vi "MD5 PaddingU8.vi"(10 "Pre Buffer Size":i64, 11 "Current Buffer":u8[](array[numeric])) -> (3 "MD5 Padded Buffer":u8[](array[numeric]))   [LabVIEW 2009]
doc: "A U8 padding VI for MD5 hash generation"
panel:
  # "[OpenG VI Tags] ***Do Not Remove***"
  # "MD5 Padding.vi\n\nDerived from the RSA Data Security, Inc. MD5 Message-Digest Algorithm\n\nPlease visit http://www.OpenG.org to learn about the\nOpen Source LabVIEW software movement.\n\nNOTICE -- YOU MUST LEAVE THIS NOTICE IN PLACE.  PER THE TERMS OF THE LICENSE BELOW, YOU MAY SUBLICENSE THIS SOFTWARE \nIN ANY WAY THAT DOES NOT CONFLICT WITH THIS LICENSE.\n\n### BSD License (http://www.opensource.org/licenses/bsd-license.php) Begin ###\n \nCopyright (c) 2004, Enrique Vargas <vargas@visecurity.com>\n\nAll rights reserved.\n\nRedistribution and use in source and binary forms, with or without modification, are permitted provided that the following conditions are met:\n\n    * Redistributions of source code must retain the above copyright notice, this list of conditions and the following disclaimer.\n    * Redistributions in binary form must reproduce the above copyright notice, this list of conditions and the following disclaimer in the \n       documentation and/or other materials provided with the distribution.\n    * Neither the name of SciWare, James Kring, Inc., nor the names of its contributors may be used to endorse or promote products derived \n       from this software without specific prior written permission.\n\nTHIS SOFTWARE IS PROVIDED BY THE COPYRIGHT HOLDERS AND CONTRIBUTORS \"AS IS\" AND ANY EXPRESS OR IMPLIED WARRANTIES, \nINCLUDING, BUT NOT LIMITED TO, THE IMPLIED WARRANTIES OF MERCHANTABILITY AND FITNESS FOR A PARTICULAR PURPOSE ARE \nDISCLAIMED. IN NO EVENT SHALL THE COPYRIGHT OWNER OR CONTRIBUTORS BE LIABLE FOR ANY DIRECT, INDIRECT, INCIDENTAL,\n SPECIAL, EXEMPLARY, OR CONSEQUENTIAL DAMAGES (INCLUDING, BUT NOT LIMITED TO, PROCUREMENT OF SUBSTITUTE GOODS OR \nSERVICES; LOSS OF USE, DATA, OR PROFITS; OR BUSINESS INTERRUPTION) HOWEVER CAUSED AND ON ANY THEORY OF LIABILITY, \nWHETHER IN CONTRACT, STRICT LIABILITY, OR TORT (INCLUDING NEGLIGENCE OR OTHERWISE) ARISING IN ANY WAY OUT OF THE USE \nOF THIS SOFTWARE, EVEN IF ADVISED OF THE POSSIBILITY OF SUCH DAMAGE.\n\n### BSD License End ###"
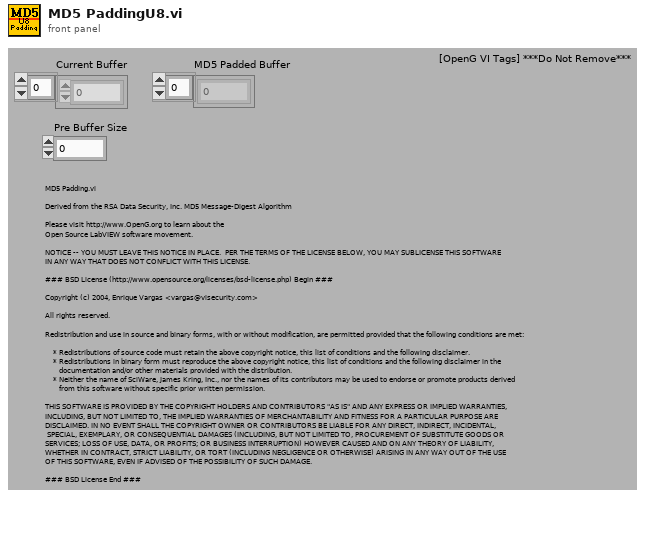
[diagram p1: front panel]
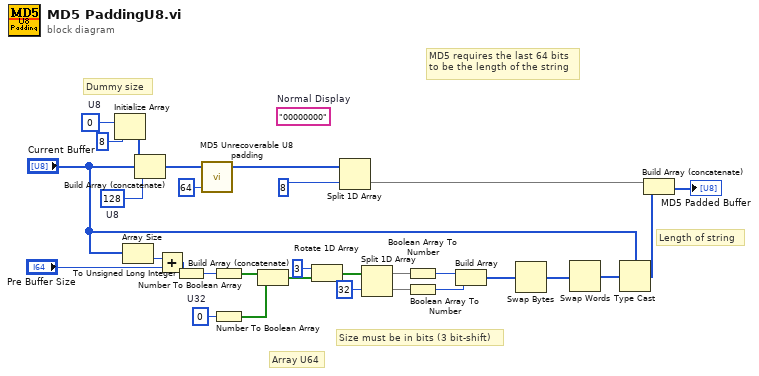
[diagram p0: block diagram]
diagram:
  w7 = u8 0  # U8
  w9 = u8 128  # U8
  w27 = u32 0  # U32
  (unwired) "00000000"  # Normal Display
  # "Size must be in bits (3 bit-shift)"
  # "Dummy size"
  # "Array U64"
  # "Length of string"
  # "MD5 requires the last 64 bits\nto be the length of the string"
  n1 = Initialize Array(w7, 8 ("dimension size")) -> (w8:u8[])
  n2 = Array Size(array="Current Buffer") -> (size(s)=w15:i32)
  n3 = Build Array (concatenate)(w8, "Current Buffer", w9) -> (w10:u8[])
  n4 = Add(x=w15, y="Pre Buffer Size") -> (x+y=w13:i64)
  n5 = To Unsigned Long Integer(number=w13) -> (unsigned 32bit integer=w28:u32)
  n6 = call "MD5 Unrecoverable U8 padding.vi"("Block Size (16)"=64, "Message"=w10) -> ("Padded message"=w5:u8[])  [unwired: 3 in]
  n7 = Number To Boolean Array(number=w28) -> (Boolean array=w26:bool[])
  n8 = Number To Boolean Array(number=w27) -> (Boolean array=w25:bool[])
  n9 = Build Array (concatenate)(w26, w25) -> (w24:bool[])
  n10 = Rotate 1D Array(1:w24, 2:3 ("n")) -> (0:w22:bool[])
  n11 = Split 1D Array(array=w5, index=8 ("offset (0)")) -> (second subarray=w3:u8[])  [unwired: 1 out]
  n12 = Split 1D Array(array=w22, index=32) -> (first subarray=w20:bool[], second subarray=w19:bool[])
  n13 = Boolean Array To Number(Boolean array=w20) -> (number=w18:u32)
  n14 = Boolean Array To Number(Boolean array=w19) -> (number=w17:u32)
  n15 = Build Array(w18, w17) -> (w16:u32[])
  n16 = Swap Bytes(anything=w16) -> (byte swapped=w30:u32[])
  n17 = Swap Words(1:w30) -> (0:w29:u32[])
  n18 = Type Cast(type="Current Buffer", x=w29) -> (*(type *) &x=w1:u8[])
  n19 = Build Array (concatenate)(w3, w1) -> (→"MD5 Padded Buffer":u8[])
